vi "Create.vi"(7 "Direction":T1, 8 "error in (no error)":errorcluster, 9 "Custom Config Data":u8[](array[numeric]), 10 "Name":string, 11 "CIFTag in":refnum<class "CIFTagDouble.lvclass">) -> (0 "error out":errorcluster, 3 "CIFTag out":refnum<class "CIFTagDouble.lvclass">)   [LabVIEW 2021, in "CIFTagDouble.lvclass"]
uses:
  CIFTagDouble.lvclass
  D:/dev/CIF-LVCore/src/Channels/CIFChannels/CIFChannels.lvclass
  D:/dev/CIF-LVCore/src/Channels/CIFTag/CIFTag/CIFTag.lvclass
  CIFChannels/Typedef/Direction.ctl
  CIFChannels/Typedef/Disconnect Behavior.ctl
  CIFChannels/CIFChannels.lvclass/CIFChannels.ctl
  CIFChannels/Typedef/Channel State.ctl
  CIFTagDouble.lvclass/CIFTagDouble.ctl
  CIFTag/CIFTag.lvclass/CIFTag.ctl
  5c81bccc-e622-4fe9-9720-12299560a745.vi
  522c0ff3-de7b-4614-b37e-c276d07c7241.vi
  05c6e502-0377-480c-a15d-085597602460.vi
  730ee9f7-183b-45cd-9827-7f858eceece4.vi
  CIFChannels/Accessors/Write Channel State.vi
  CIFTag/Accessors/Write CIF Channel.vi
  CIFChannels/SubVIs/Get Type from Class.vi
  CIFChannels/Accessors/Write Type.vi
  CIFChannels/Accessors/Write Channel Class.vi
  CIFChannels/Accessors/Write Direction.vi
  CIFChannels/Accessors/Write Disconnect Behavior.vi
  CIFChannels/Accessors/Write Name.vi
  CIFChannels/Accessors/Write Custom Config Data.vi
  <vilib>/CIFChannels/SubVIs/Add Error.vi
  5c81bccc-e622-4fe9-9720-12299560a745.vi/c28b0ead-42ad-4072-80a2-aca7f2bd7ce3.vi
  <vilib>/CIFChannels/SubVIs/Get dll Path.vi
  522c0ff3-de7b-4614-b37e-c276d07c7241.vi/4bc1c15b-36ab-481f-b8dd-c64075ce723a.vi
  522c0ff3-de7b-4614-b37e-c276d07c7241.vi/d83cb72b-7713-41fc-a3d1-682de79cf574.vi
  05c6e502-0377-480c-a15d-085597602460.vi/c28b0ead-42ad-4072-80a2-aca7f2bd7ce3.vi
  730ee9f7-183b-45cd-9827-7f858eceece4.vi/4bc1c15b-36ab-481f-b8dd-c64075ce723a.vi
  <vilib>/CIFChannels/SubVIs/Append Error Location.vi
  <vilib>/Utility/LVClass/Get LV Class Name.vi
  CIFChannels/CIFChannels.lvclass
panel:
  out "error out 2":errorcluster
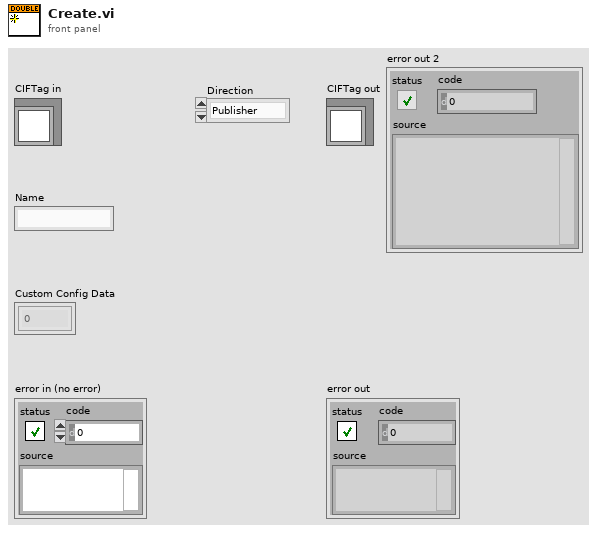
[diagram p1: front panel]
types:
  T1 = typedef "CIFChannels.lvclass/Direction.ctl" = enum16{"Publisher", "Subscriber"}
  T2 = typedef "CIFChannels.lvclass/Disconnect Behavior.ctl" = enum16{"Default value", "Last value", "Error with default"}
  T3 = typedef "CIFChannels.lvclass/Channel State.ctl" = enum16{"Creating", "Disconnected", "Connecting", "Connected", "Destroyed"}
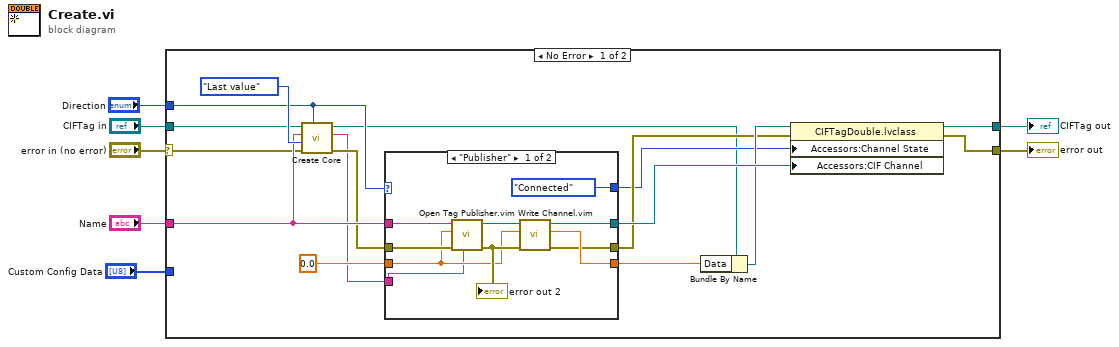
[diagram p0: block diagram]
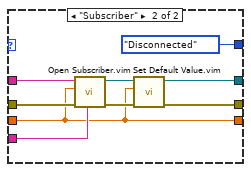
[diagram p2: hidden frame]
diagram:
  n1 = case shown="No Error" "error in (no error)" {
    selector: "error in (no error)" -> [w12 w44]
    tunnel: [w22 w44] -> w6
    tunnel: [w16 w43] -> w4
    tunnel: "CIFTag in" -> [w11 w43]
    tunnel: "Name" -> [w21 _]
    tunnel: "Direction" -> [w15 _]
    tunnel: "Custom Config Data" -> [_ _]
    frame No Error {
      n2 = call "Create Core.vi"("Direction"=w15, "error in (no error)"=w12, "Disconnect Behavior"=Disconnect_Behavior."Last value", "Name"=w21, "CIFChannels in"=w11) -> ("error out"=w10:errorcluster, "Channel Type"=w8:string, "CIFChannels out"=w9:refnum<class "CIFTagDouble.lvclass">)  [unwired: 4 in]
      n3 = case shown="\"Publisher\"" w15 {
        tunnel: w21 -> [w33 w41]
        tunnel: w10 -> [w32 w40]
        tunnel: [w29 w37] -> w20
        tunnel: 0.0 ("Default Value") -> [w28 w34]
        tunnel: [w27 w34] -> w18
        tunnel: [w26 w36] -> w17
        tunnel: w8 -> [w25 w35]
        tunnel: [Channel_State."Connected" ("Channel State") Channel_State."Disconnected" ("Channel State")] -> w14
        frame "Publisher" {
          n4 = call "Open Tag Publisher.vim"("Channel Type Description"=w25, "error in"=w32, "Input Type"=w28, "Channel Name"=w33) -> ("error out"=w30:errorcluster, "CIF Channel"=w31:refnum<k21>)  [unwired: 6 in]
          "error out 2" <- w30
          n5 = call "Write Channel.vim"("error in"=w30, "Data in"=w28, "CIF Channel in"=w31) -> ("error out"=w26:errorcluster, "Data out"=w27:dbl, "CIF Channel out"=w29:refnum<k21>)  [unwired: 5 in, 1 out]
        }
        frame "Subscriber" {
          n6 = call "Open Subscriber.vim"("Channel Type Description"=w35, "error in"=w40, "Input Type"=w34, "Channel Name"=w41) -> ("error out"=w39:errorcluster, "CIF Channel"=w38:refnum<k21>)  [unwired: 6 in]
          n7 = call "Set Default Value.vim"("error in"=w39, "Data in"=w34, "CIF Channel in"=w38) -> ("error out"=w36:errorcluster, "CIF Channel out"=w37:refnum<k21>)  [unwired: 7 in]
        }
      }
      n8 = Bundle By Name(cluster=w9, "Data"=w18) -> (w19:refnum<class "CIFTagDouble.lvclass">)
      n9 = property class="CIFTagDouble.lvclass"(reference=w19, error in=w17, "Accessors:Channel State"=w14, "Accessors:CIF Channel"=w20) -> (reference out=w16:refnum<class "CIFTagDouble.lvclass">, error out=w22:errorcluster)
    }
    frame Error {
    }
  }
  "error out" <- w6
  "CIFTag out" <- w4
